vi "Array to Graph.vi"(1 "Y Index":i32, 2 "X Index":i32, 3 "Input 2-D Array":dbl[][](array[numeric]) format="%.2f") -> (0 "Output Cluster to Graph":cluster{dbl[], dbl[]} {"?" format="%.2f"; "?" format="%.2f"})   [LabVIEW 2016]
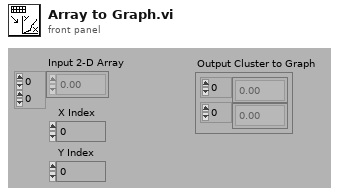
[diagram p1: front panel]
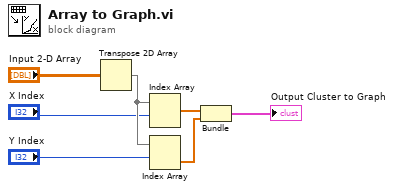
[diagram p0: block diagram]
diagram:
  n1 = Transpose 2D Array(2D array="Input 2-D Array") -> (transposed array=w7:dbl[][])
  n2 = Index Array(array=w7, index (row)="X Index") -> (element=w2:dbl[])  [unwired: 1 in]
  n3 = Index Array(array=w7, index (row)="Y Index") -> (element=w3:dbl[])  [unwired: 1 in]
  n4 = Bundle(w2, w3) -> (→"Output Cluster to Graph":cluster{dbl[], dbl[]})  [unwired: 1 in]
